vi "Actuators Get Moving.vi"(0 "Notifier Name":string, 11 "Error In":errorcluster) -> (4 "Notifier Name Out":string, 8 "Moving":bool[](array[boolean]), 15 "Error Out":errorcluster)   [LabVIEW 2020]
uses:
  Actuators Controls/Actuators Note Type.ctl
  Actuators Controls/Actuators Actions.ctl
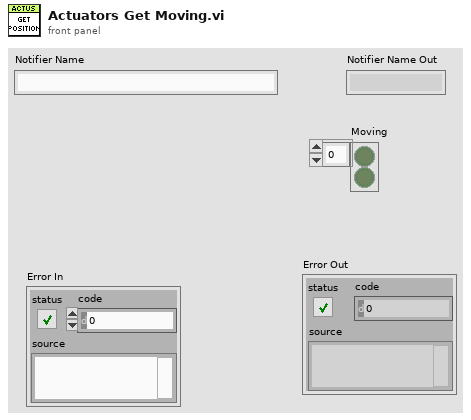
[diagram p1: front panel]
types:
  T1 = typedef "Actuators Note Type.ctl" = cluster{"Actions":T2, "Cmd Received ":bool, "Setpoint":dbl[], "Position":dbl[], "Channel":i32[], "Jog Step":dbl[], "Velocity":dbl[], "Acceleration":dbl[], "Status Bits":u32[], "Moving":bool[]}
  T2 = typedef "Actuators Actions.ctl" = enum16{"Nothing", "Get Position", "Get Acceleration", "Get Velocity", "Get Jog Step", "Set Acceleration", "Set Velocity", "Set Jog Step", "Move Absolute", "Move Relative", "Jog Forward", "Jog Reverse", "Set Moving", "Halt", "Quit"}
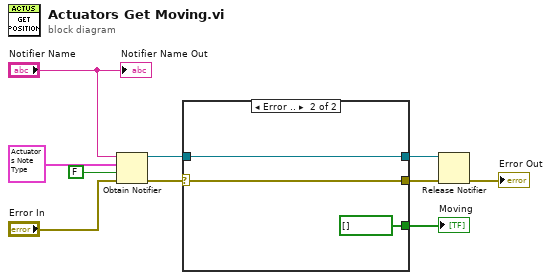
[diagram p0: block diagram]
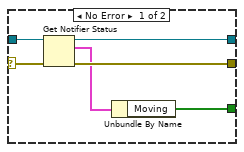
[diagram p2: hidden frame]
diagram:
  n1 = Obtain Notifier(name (unnamed)="Notifier Name", notification data type=T1 {"Actions"=enum."Nothing", "Cmd Received "=FALSE, "Setpoint"=[], "Position"=[], "Channel"=[], "Jog Step"=[], "Velocity"=[], "Acceleration"=[], "Status Bits"=[], "Moving"=[]} ("Actuators Note"), create if not found? (T)=FALSE, error in (no error)="Error In") -> (notifier out=w6:refnum<notifier>, error out=w9:errorcluster)  [unwired: 1 out]
  n2 = case shown="Error .." w9 {
    selector: w9 -> [w15 w18]
    tunnel: w6 -> [w16 w19]
    tunnel: [w14 w19] -> w5
    tunnel: [w13 w18] -> w4
    tunnel: [w11 bool[] [] ("Moving")] -> w1
    frame No Error {
      n3 = Get Notifier Status(notifier=w16, error in (no error)=w15) -> (notifier out=w14:refnum<notifier>, current notification=w12:T1, error out=w13:errorcluster)  [unwired: 2 out]
      n4 = Unbundle By Name(w12) -> ("Moving"=w11:bool[])
    }
    frame Error {
    }
  }
  "Moving" <- w1
  n5 = Release Notifier(notifier=w5, error in (no error)=w4) -> (error out=→"Error Out":errorcluster)  [unwired: 1 in, 2 out]
  "Notifier Name Out" <- "Notifier Name"
